vi "GetIdentity.vi"(8 "error in (no error)":errorcluster, 11 "SMO in":refnum<class "SMO.lvclass">) -> (0 "error out":errorcluster, 1 "GUID":string, 2 "Name":string, 3 "SMO out":refnum<class "SMO.lvclass">)   [LabVIEW 2021, in "smo.lvlib" / "SMO.lvclass"]
uses:
  SMO.lvclass
  Support/Attribute.Identity/Attribute.Identity.lvclass
  SMO.lvclass/SMO.ctl
  Support/Attribute.Identity/Attribute.Identity.lvclass/Attribute.Identity.ctl
  ReftoDVR--SMO.vi
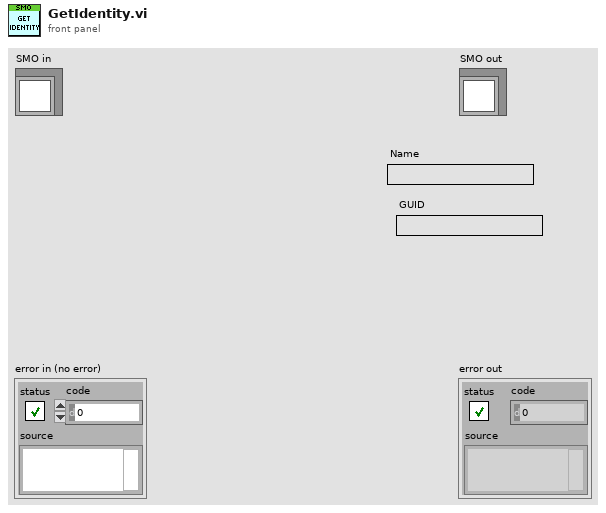
[diagram p1: front panel]
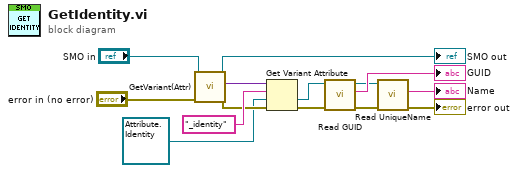
[diagram p0: block diagram]
diagram:
  n1 = call "GetVariant(Attr).vi"("error in (no error)"="error in (no error)", "SMO in"="SMO in") -> ("error out"=w10:errorcluster, "[Attributes]"=w12:variant, "SMO out"=→"SMO out":refnum<class "SMO.lvclass">)  [unwired: 7 in]
  n2 = Get Variant Attribute(Variant=w12, name="_identity", default value (empty Variant)=refnum<class "Attribute.Identity.lvclass"> refnum, error in=w10) -> (value=w4:refnum<class "Attribute.Identity.lvclass">, error out=w5:errorcluster)  [unwired: 2 out]
  n3 = call "Read GUID.vi"("error in (no error)"=w5, "Attribute.Identity in"=w4) -> ("error out"=→"error out":errorcluster, "GUID"=→"GUID":string, "Attribute.Identity out"=w3:refnum<class "Attribute.Identity.lvclass">)  [unwired: 7 in]
  n4 = call "Read UniqueName.vi"("Attribute.Identity in"=w3) -> ("Unique Name"=→"Name":string)  [unwired: 9 in, 1 out]
